vi "ITX Folder to TDMS.vi"(8 "error in (no error)":errorcluster, 11 "Folder Path":path) -> (0 "error out":errorcluster)   [LabVIEW 2016]
panel:
  in  "Single File?":bool
  out "Elapsed Time (s)":dbl
  out "Numeric":i32
  # "T = Create 1 TDMS file for the entire folder\nF = Create 1 TDMS file for each ITX file"
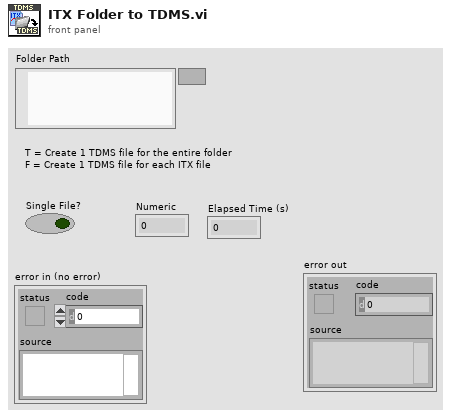
[diagram p1: front panel]
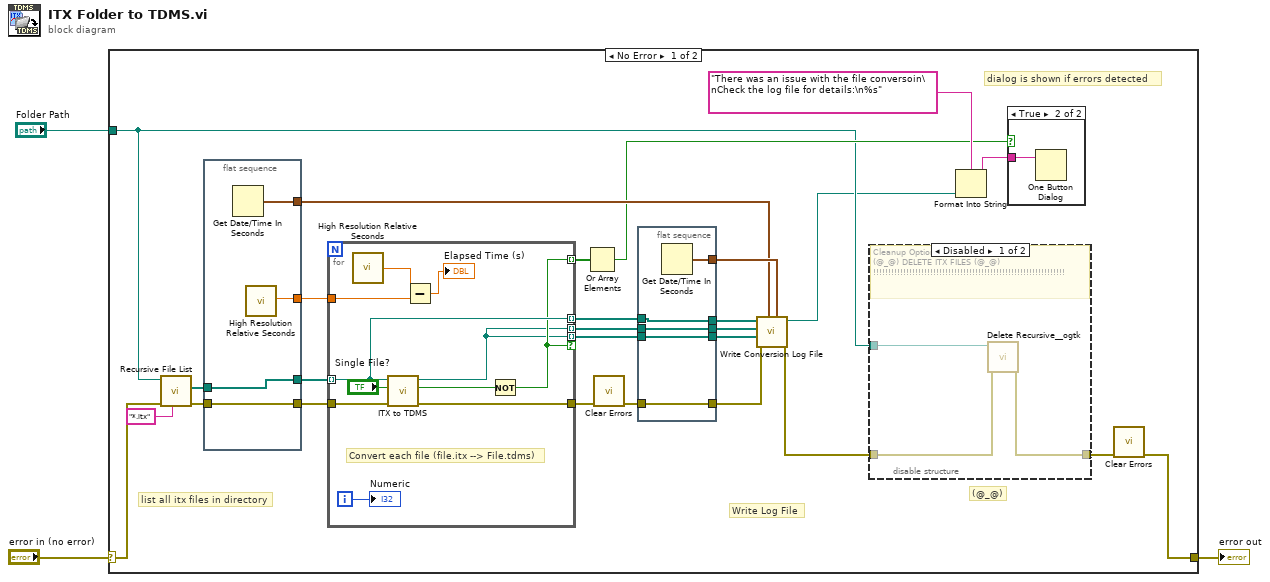
[diagram p0: block diagram]
diagram:
  n1 = case shown="No Error" "error in (no error)" {
    selector: "error in (no error)" -> [w29 w56]
    tunnel: [w4 w56] -> w2
    tunnel: "Folder Path" -> [w7 _]
    frame No Error {
      # "(@_@)"
      # "dialog is shown if errors detected"
      # "list all itx files in directory"
      # "Write Log File"
      n2 = call <vilib>:"Recursive File List.vi"("pattern"="*.itx", "error in (no error)"=w29, "Folder Path"=w7) -> ("error out"=w25:errorcluster, "All Files in Dir"=w24:path[])  [unwired: 4 in, 3 out]
      n3 = flat-sequence {
        tunnel: [w39] -> w28
        tunnel: [w38] -> w26
        tunnel: w25 -> [w38]
        tunnel: w24 -> [w37]
        tunnel: [w37] -> w23
        tunnel: [w36] -> w11
        frame #0 {
          n4 = Get Date/Time In Seconds() -> (seconds since 1Jan1904=w36:timestamp)
          n5 = call <vilib>:"High Resolution Relative Seconds.vi"() -> ("relative seconds"=w39:dbl)
        }
      }
      n6 = for {
        tunnel: w23 -> [w49] mode=indexing
        tunnel: w26 -> [w54]
        tunnel: [w53] -> w18
        tunnel: w28 -> [w50]
        tunnel: [w45] -> w19 mode=indexing if=w47
        tunnel: [w45] -> w21 mode=indexing
        tunnel: [w49] -> w22 mode=indexing
        tunnel: [w47] -> w27 mode=indexing
        i -> [w52]
        # "Convert each file (file.itx --> File.tdms)"
        n7 = call <vilib>:"High Resolution Relative Seconds.vi"() -> ("relative seconds"=w51:dbl)
        n8 = call "ITX to TDMS.vi"("error in (no error)"=w54, "Single File?"="Single File?", "file (use dialog)"=w49) -> ("error out"=w53:errorcluster, "Equal?"=w48:bool, "path out"=w45:path)  [unwired: 6 in]
        n9 = Subtract(x=w51, y=w50) -> (x-y=→"Elapsed Time (s)":dbl)
        n10 = Not(x=w48) -> (.not. x?=w47:bool)
        "Numeric" <- w52
      }
      n11 = Or Array Elements(Boolean array=w27) -> (logical OR=w8:bool)
      n12 = call <vilib>:"Clear Errors.vi"("error in (no error)"=w18) -> ("error out"=w5:errorcluster)  [unwired: 5 in, 1 out]
      n13 = flat-sequence {
        tunnel: w22 -> [w34]
        tunnel: [w35] -> w13
        tunnel: w21 -> [w35]
        tunnel: [w34] -> w14
        tunnel: [w33] -> w20
        tunnel: w19 -> [w33]
        tunnel: w5 -> [w32]
        tunnel: [w32] -> w9
        tunnel: [w31] -> w17
        frame #0 {
          n14 = Get Date/Time In Seconds() -> (seconds since 1Jan1904=w31:timestamp)
        }
      }
      n15 = call "Write Conversion Log File.vi"("End time"=w17, "Start time"=w11, "error in (no error)"=w9, "Failed Converted Files"=w20, "Converted Files"=w13, "Original Files"=w14) -> ("error out"=w10:errorcluster, "Log File Path"=w6:path)  [unwired: 4 in]
      n16 = disable-structure shown="Disabled" {
        disable-tunnel: w10 -> [w42 w43]
        disable-tunnel: [w41 w43] -> w12
        disable-tunnel: w7 -> [w40 _]
        frame Disabled {
          # "Cleanup Option:\n(@_@) DELETE ITX FILES (@_@)\n!!!!!!!!!!!!!!!!!!!!!!!!!!!!!!!!!!!!!!!!!!!!!!!!!!!!!!!!!!!!!!!!"
          n17 = call <userlib>:"Delete Recursive__ogtk.vi"("error in (no error)"=w42, "Path"=w40) -> ("error out"=w41:errorcluster)  [unwired: 8 in, 1 out]
        }
        frame Enabled {
        }
      }
      n18 = Format Into String(format string="There was an issue with the file conversoin\nCheck the log file for details:\n%s", w6) -> (resulting string=w16:string)  [unwired: 2 in, 1 out]
      n19 = case shown="True" w8 {
        tunnel: w16 -> [_ w55]
        frame False {
        }
        frame True {
          n20 = One Button Dialog(message=w55) -> ()  [unwired: 1 in, 1 out]
        }
      }
      n21 = call <vilib>:"Clear Errors.vi"("error in (no error)"=w12) -> ("error out"=w4:errorcluster)  [unwired: 5 in, 1 out]
    }
    frame Error {
    }
  }
  "error out" <- w2
